vi "To XML.vi"(8 "error in (no error)":errorcluster, 9 "Parent":refnum<k20>, 10 "Document":refnum<k20>, 11 "Package in":refnum<class "Package.lvclass">) -> (0 "error out":errorcluster)   [LabVIEW 2017, in "Cobertura.lvlib" / "Package.lvclass"]
uses:
  Package.lvclass
  Package.lvclass/Package.ctl
  Class/Class.lvclass
  <resource>/objmgr/DOMUserDefRef.rc
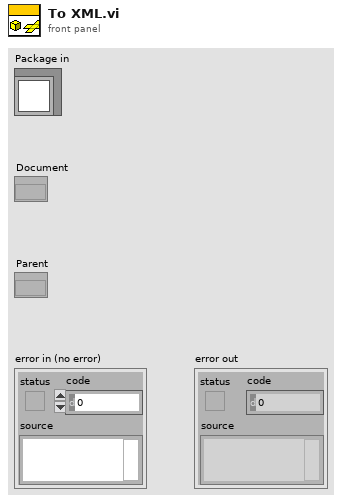
[diagram p1: front panel]
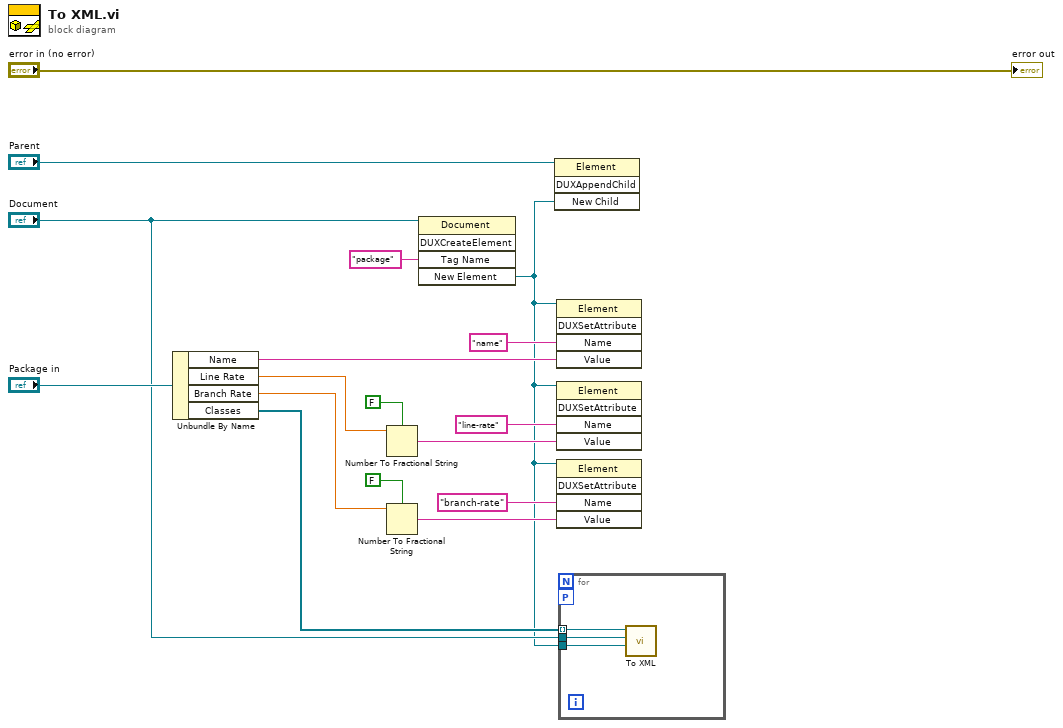
[diagram p0: block diagram]
diagram:
  n1 = Unbundle By Name("Package in") -> ("Name"=w8:string, "Line Rate"=w7:dbl, "Branch Rate"=w6:dbl, "Classes"=w4:refnum<class "Class.lvclass">[])
  n2 = Number To Fractional String(use system decimal point (T)=FALSE, number=w7) -> (F-format string=w14:string)  [unwired: 2 in]
  n3 = Number To Fractional String(use system decimal point (T)=FALSE, number=w6) -> (F-format string=w10:string)  [unwired: 2 in]
  n4 = invoke class="Document" method="DUXCreateElement"(reference="Document", "Tag Name"="package") -> ("New Element"=w1:refnum<k20>)  [unwired: 3 in, 4 out]
  n5 = invoke class="Element" method="DUXAppendChild"(reference="Parent", "New Child"=w1) -> ()  [unwired: 2 in, 4 out]
  n6 = invoke class="Element" method="DUXSetAttribute"(reference=w1, "Name"="name", "Value"=w8) -> ()  [unwired: 2 in, 5 out]
  n7 = invoke class="Element" method="DUXSetAttribute"(reference=w1, "Name"="line-rate", "Value"=w14) -> ()  [unwired: 2 in, 5 out]
  n8 = invoke class="Element" method="DUXSetAttribute"(reference=w1, "Name"="branch-rate", "Value"=w10) -> ()  [unwired: 2 in, 5 out]
  n9 = for {
    tunnel: w4 -> [w20] mode=indexing
    tunnel: "Document" -> [w19]
    tunnel: w1 -> [w18]
    workers-P: _ -> [_]
    n10 = call-dynamic "To XML.vi"("Parent"=w18, "Document"=w19, "Class in"=w20) -> ()  [unwired: 8 in, 1 out]
  }
  "error out" <- "error in (no error)"
